vi "HomeZero.vi"   [LabVIEW 2015]
uses:
  <userlib>/Newport ESP301/Newport ESP301.lvlib
types:
  T1 = enum16{"Find +0 Position Count", "Find Home and Index Signals", "Find Home Signal", "Find Positive Limit Signal", "Find Negative Limit Signal", "Find Positve Limit and Index Signals", "Find Negative Limit and Index Signals"}
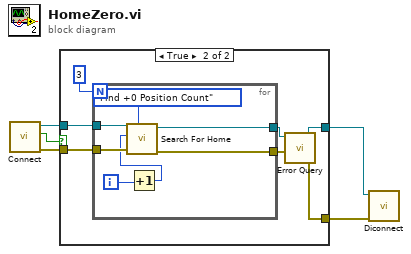
[diagram p0: block diagram]
diagram:
  n1 = call "Connect.vi"() -> ("error out"=w4:errorcluster, "Connected"=w3:bool, "VISA resource name out"=w5:refnum<visa-resource-name>)  [unwired: 5 in]
  n2 = case shown="True" w3 {
    tunnel: w5 -> [w7 w14]
    tunnel: w4 -> [w6 w13]
    tunnel: [w7 w9] -> w2
    tunnel: [w6 w8] -> w1
    frame False {
    }
    frame True {
      n3 = for {
        N: 3 -> [_]
        tunnel: w14 -> [w21]
        tunnel: w13 -> [w20]
        tunnel: [w16] -> w11
        tunnel: [w15] -> w10
        i -> [w19]
        n4 = Increment(x=w19) -> (x+1=w18:i32)
        n5 = call <userlib>:"Search For Home.vi"("Home mode"=T1."Find +0 Position Count", "error in (no error)"=w20, "Axis (1)"=w18, "VISA resource name"=w21) -> ("error out"=w15:errorcluster, "VISA resource name out"=w16:refnum<visa-resource-name>)  [unwired: 3 in]
      }
      n6 = call <userlib>:"Error Query.vi"("error in (no error)"=w10, "VISA resource name"=w11) -> ("error out"=w8:errorcluster, "VISA resource name out"=w9:refnum<visa-resource-name>)  [unwired: 2 in, 2 out]
    }
  }
  n7 = call "Diconnect.vi"("error in (no error)"=w1, "VISA resource name"=w2) -> ()  [unwired: 6 in]
